vi "Cascade get an image.vi"(3 "error in":errorcluster, 4 "Image In":T1, 5 "Handles in":T2) -> (0 "error out":errorcluster, 1 "new image acquired?":bool, 2 "Image Out":T1)   [LabVIEW 2011]
doc: "Copyright (c) 2004-2006 Jeff Gelles Brandeis University"
uses:
  <vilib>/vision/Image Controls.llb/IMAQ Image.ctl
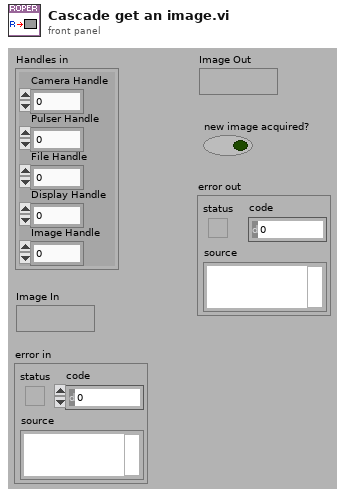
[diagram p1: front panel]
types:
  T1 = typedef "IMAQ Image.ctl" = refnum<image>
  T2 = cluster{"Camera Handle":u32, "Pulser Handle":u32, "File Handle":u32, "Display Handle":u32, "Image Handle":u32}
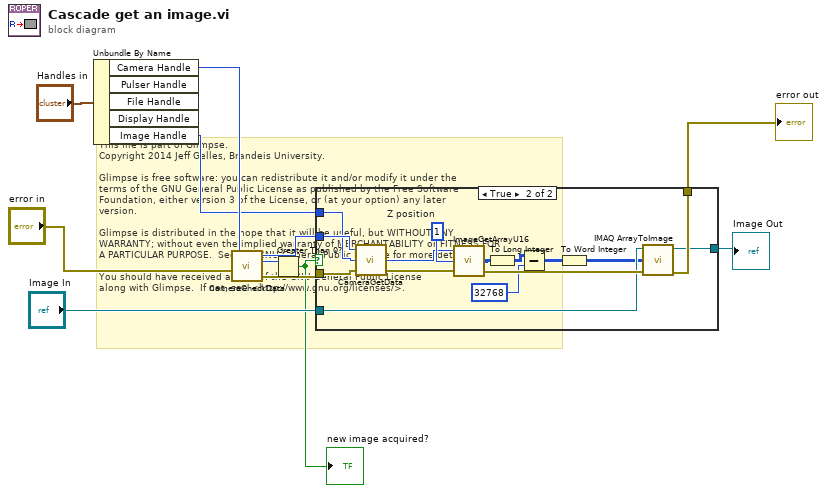
[diagram p0: block diagram]
diagram:
  # "This file is part of Glimpse. \nCopyright 2014 Jeff Gelles, Brandeis University.    \n\nGlimpse is free software: you can redistribute it and/or modify it under the \nterms of the GNU General Public License as published by the Free Software \nFoundation, either version 3 of the License, or (at your option) any later \nversion.\n\nGlimpse is distributed in the hope that it will be useful, but WITHOUT ANY \nWARRANTY; without even the implied warranty of MERCHANTABILITY or FITNESS FOR \nA PARTICULAR PURPOSE.  See the GNU General Public License for more details.\n\nYou should have received a copy of the GNU General Public License\nalong with Glimpse.  If not, see <http://www.gnu.org/licenses/>."
  n1 = Unbundle By Name("Handles in") -> ("Camera Handle"=w6:u32, "Image Handle"=w5:u32)  [unwired: 3 out]
  n2 = call <userlib>:"CameraCheckData.vi"("Camera Handle"=w6, "error in"="error in") -> ("Camera Handle"=w2:u32, "Number Of Frames Available"=w3:i32, "error out"=w4:errorcluster)
  n3 = Greater Than 0?(x=w3) -> (x > 0?=w1:bool)
  "new image acquired?" <- w1
  n4 = case shown="True" w1 {
    tunnel: w2 -> [_ w28]
    tunnel: w4 -> [w13 w27]
    tunnel: w5 -> [_ w25]
    tunnel: "Image In" -> [w12 w20]
    tunnel: [w13 w19] -> w10
    tunnel: [w12 w18] -> w11
    frame False {
    }
    frame True {
      w24 = u32 1  # Z position
      n5 = call <userlib>:"CameraGetData.vi"("error in"=w27, "Data Handle"=w25, "Camera Handle"=w28) -> ("error out"=w26:errorcluster, "Data Handle"=w23:u32)  [unwired: 1 out]
      n6 = call <userlib>:"ImageGetArrayU16.vi"("error in"=w26, "Z position"=w24, "Image Handle"=w23) -> ("error out"=w22:errorcluster, "Array uint 16"=w21:u16[][])  [unwired: 1 out]
      n7 = To Long Integer(number=w21) -> (32bit integer=w16:i32[][])
      n8 = Subtract(x=w16, y=32768 ("values")) -> (x-y=w17:i32[][])
      n9 = To Word Integer(number=w17) -> (16bit integer=w14:i16[][])
      n10 = call "IMAQ ArrayToImage"("error in (no error)"=w22, "Image Pixels (I16)"=w14, "Image"=w20) -> ("error out"=w19:errorcluster, "Image Out"=w18:T1)  [unwired: 3 in, 4 out]
    }
  }
  "Image Out" <- w11
  "error out" <- w10
